vi "test_Multiple Writes and Reads.vi"(8 "error in (no error)":errorcluster, 11 "Scalar Channels Testing in":refnum<class "FPGA Addon Test Class.lvclass">) -> (0 "error out":errorcluster, 3 "Scalar Channels Testing out":refnum<class "FPGA Addon Test Class.lvclass">)   [LabVIEW 2019]
uses:
  FPGA Addon Test Class.lvclass
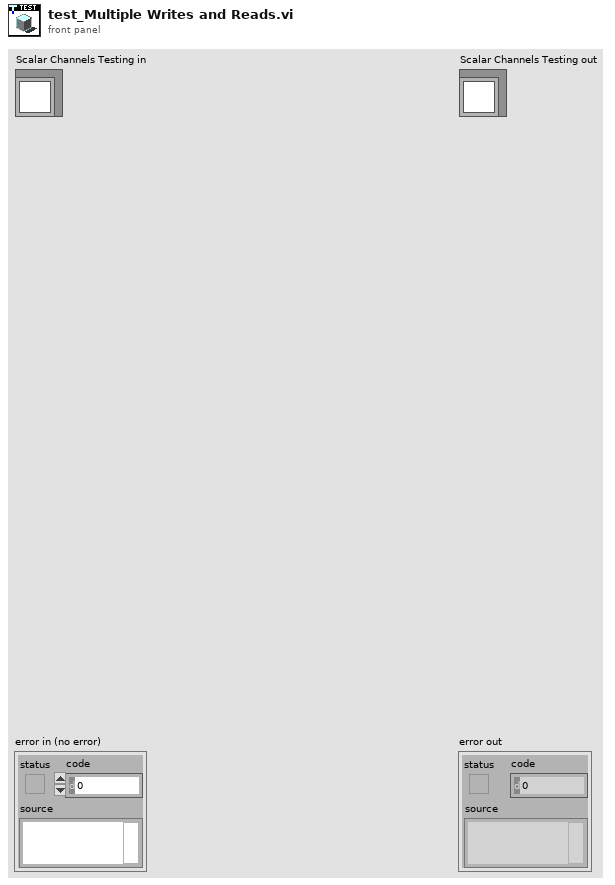
[diagram p1: front panel]
types:
  T1 = typedef "NI_VS Workspace ExecutionAPI.lvlib/WorkspaceAPI.ctl" = refnum<k24>
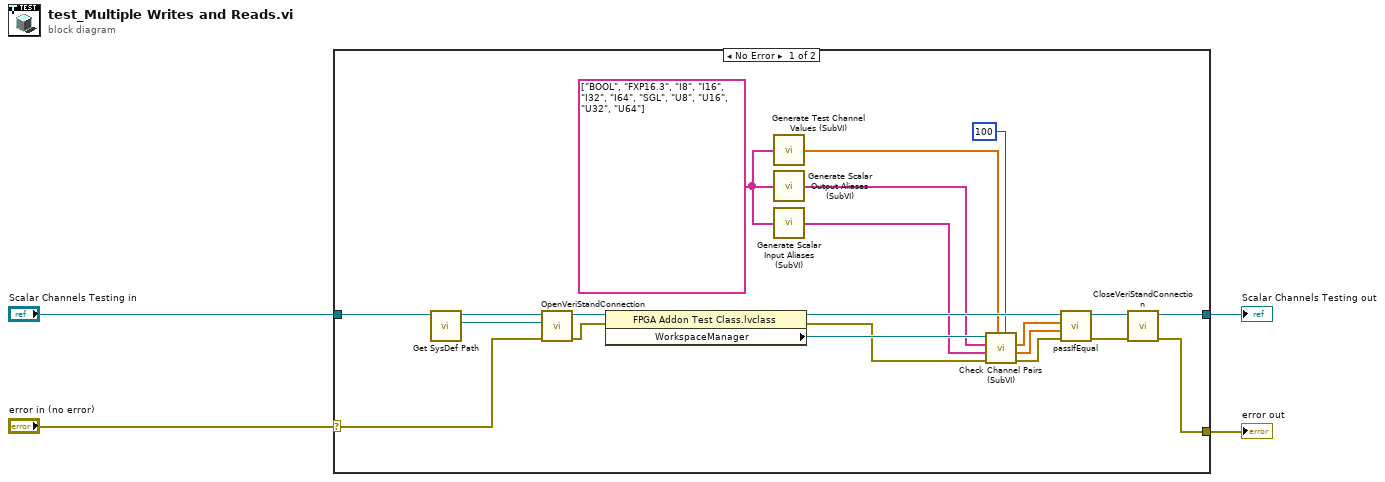
[diagram p0: block diagram]
diagram:
  n1 = case shown="No Error" "error in (no error)" {
    selector: "error in (no error)" -> [w6 w27]
    tunnel: [w24 w27] -> w3
    tunnel: [w25 w26] -> w1
    tunnel: "Scalar Channels Testing in" -> [w7 w26]
    frame No Error {
      w20 = string[] ["BOOL", "FXP16.3", "I8", "I16", "I32", "I64", "SGL", "U8", "U16", "U32", "U64"]
      n2 = call "Get SysDef Path.vi"("Scalar Channels Testing in"=w7) -> ("SysDef Path"=w5:path, "Scalar Channels Testing out"=w8:refnum<class "FPGA Addon Test Class.lvclass">)  [unwired: 9 in]
      n3 = call-dynamic "OpenVeriStandConnection.vi"("error in (no error)"=w6, "System Definition File"=w5, "VeriStand Test Case in"=w8) -> ("error out"=w23:errorcluster, "VeriStand Test Case out"=w22:refnum<class "FPGA Addon Test Class.lvclass">)  [unwired: 6 in, 1 out]
      n4 = property class="FPGA Addon Test Class.lvclass"(reference=w22, error in=w23) -> (reference out=w18:refnum<class "FPGA Addon Test Class.lvclass">, error out=w10:errorcluster, "WorkspaceManager"=w19:T1)
      n5 = call "Generate Test Channel Values (SubVI).vi"("Aliases in"=w20) -> ("Test Channel Values out"=w11:dbl[])
      n6 = call "Generate Scalar Output Aliases (SubVI).vi"("Aliases Seed"=w20) -> ("Scalar Output Aliases"=w15:string[])
      n7 = call "Generate Scalar Input Aliases (SubVI).vi"("Aliases Seed"=w20) -> ("Scalar Input Aliases"=w14:string[])
      n8 = call "Check Channel Pairs (SubVI).vi"("milliseconds to wait"=u32 100, "Test Values"=w11, "error in (no error)"=w10, "Scalar Input Aliases"=w14, "Scalar Output Aliases"=w15, ".NET Refnum in"=w19) -> ("error out"=w17:errorcluster, "Input Scalar Channel Values"=w12:dbl[], "Output Scalar Channel Values"=w13:dbl[])  [unwired: 2 in, 1 out]
      n9 = call-dynamic "passIfEqual.vi"("error in (no error)"=w17, "y"=w12, "x"=w13, "TestCase in"=w18) -> ("error out"=w21:errorcluster, "TestCase out"=w16:refnum<class "FPGA Addon Test Class.lvclass">)  [unwired: 6 in]
      n10 = call-dynamic "CloseVeriStandConnection.vi"("error in (no error)"=w21, "VeriStand Test Case in"=w16) -> ("error out"=w24:errorcluster, "VeriStand Test Case out"=w25:refnum<class "FPGA Addon Test Class.lvclass">)  [unwired: 8 in]
    }
    frame Error {
    }
  }
  "error out" <- w3
  "Scalar Channels Testing out" <- w1
